vi "SUB_Write_GEN4_Init_data_V2_0_1 - 88.vi"(5 "Interval Time":enum16{"10ms", "33ms", "50ms"}(ring), 7 "Mode":T3, 8 "Connection Status":T1={"MAC Address"="F8:B8:54:EF:76:8D", "cnx handle"=0, "cnx flags"=5, "Address Type"=1, "Connection Interval (ms)"=8, "Timeout(ms)"=1000, "Latency"=0, "bonding handle"=255} {"Address Type" items=["Public", "Random"]}, 9 "88 tx start":bool, 10 "PCAP zero information":T4 {"Check sum" format="%x"; "Sensor 8_L" format="%x"; "Sensor 8_H" format="%x"; "Sensor 7_L" format="%x"; "Sensor 7_H" format="%x"; "Sensor 6_L" format="%x"; "Sensor 6_H" format="%x"; "Sensor 5_L" format="%x"; "Sensor 5_H" format="%x"; "Sensor 4_L" format="%x"; "Sensor 4_H" format="%x"; "Sensor 3_L" format="%x"; "Sensor 3_H" format="%x"; "Sensor 2_L" format="%x"; "Sensor 2_H" format="%x"; "Sensor 1_L" format="%x"; "Sensor 1_H" format="%x"; "Packet ID" format="%x"}, 11 "Port-act 1":refnum<visa-resource-name>="COM8") -> (0 "88 checksum":u8, 1 "88 rx start":bool)   [LabVIEW 2015]
uses:
  Cluster Type/PCAP zero information.ctl
  Type definition/write_mode.ctl
  Lib_Bled112 toolkit/type_def/connection_status_bundle.ctl
  Lib_Bled112 toolkit/type_def/address_type.ctl
  Lib_Bled112 toolkit/ble_functions/ble_write_by_handle_uint8array.vi
panel:
  in  "Delay(ms)":u32=3
  # "=> Sensor Offset Valure"
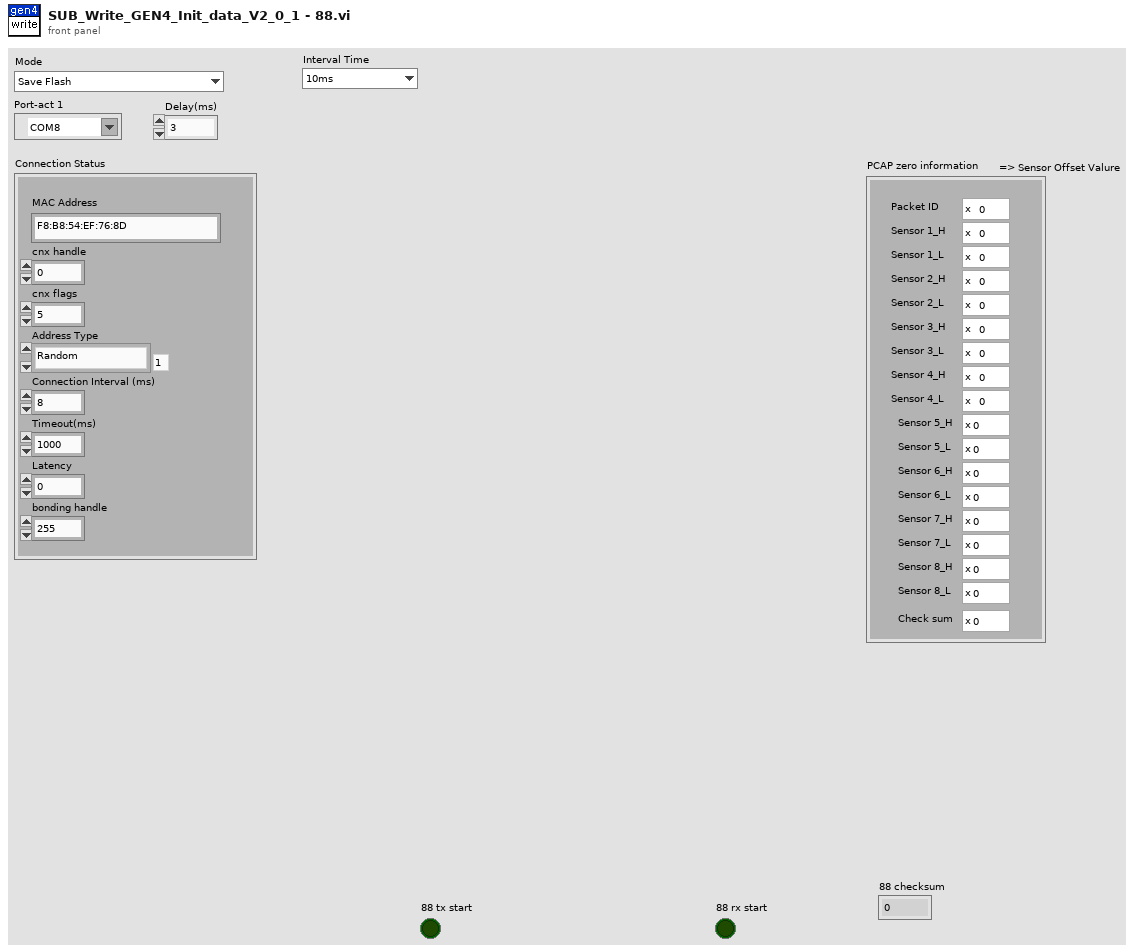
[diagram p1: front panel]
types:
  T1 = typedef "connection_status_bundle.ctl" = cluster{"MAC Address":string, "cnx handle":u8, "cnx flags":u8, "Address Type":T2, "Connection Interval (ms)":u16, "Timeout(ms)":u16, "Latency":u16, "bonding handle":u8}
  T2 = typedef "address_type.ctl" = u8
  T3 = typedef "write_mode.ctl" = enum16{"Save Flash", "Visa save", "Interval Change"}
  T4 = typedef "PCAP zero information.ctl" = cluster{"Packet ID":u8, "Sensor 1_H":u8, "Sensor 1_L":u8, "Sensor 2_H":u8, "Sensor 2_L ":u8, "Sensor 3_H":u8, "Sensor 3_L":u8, "Sensor 4_H":u8, "Sensor 4_L":u8, "Sensor 5_H":u8, "Sensor 5_L":u8, "Sensor 6_H":u8, "Sensor 6_L":u8, "Sensor 7_H":u8, "Sensor 7_L":u8, "Sensor 8_H":u8, "Sensor 8_L":u8, "Check sum":u8}
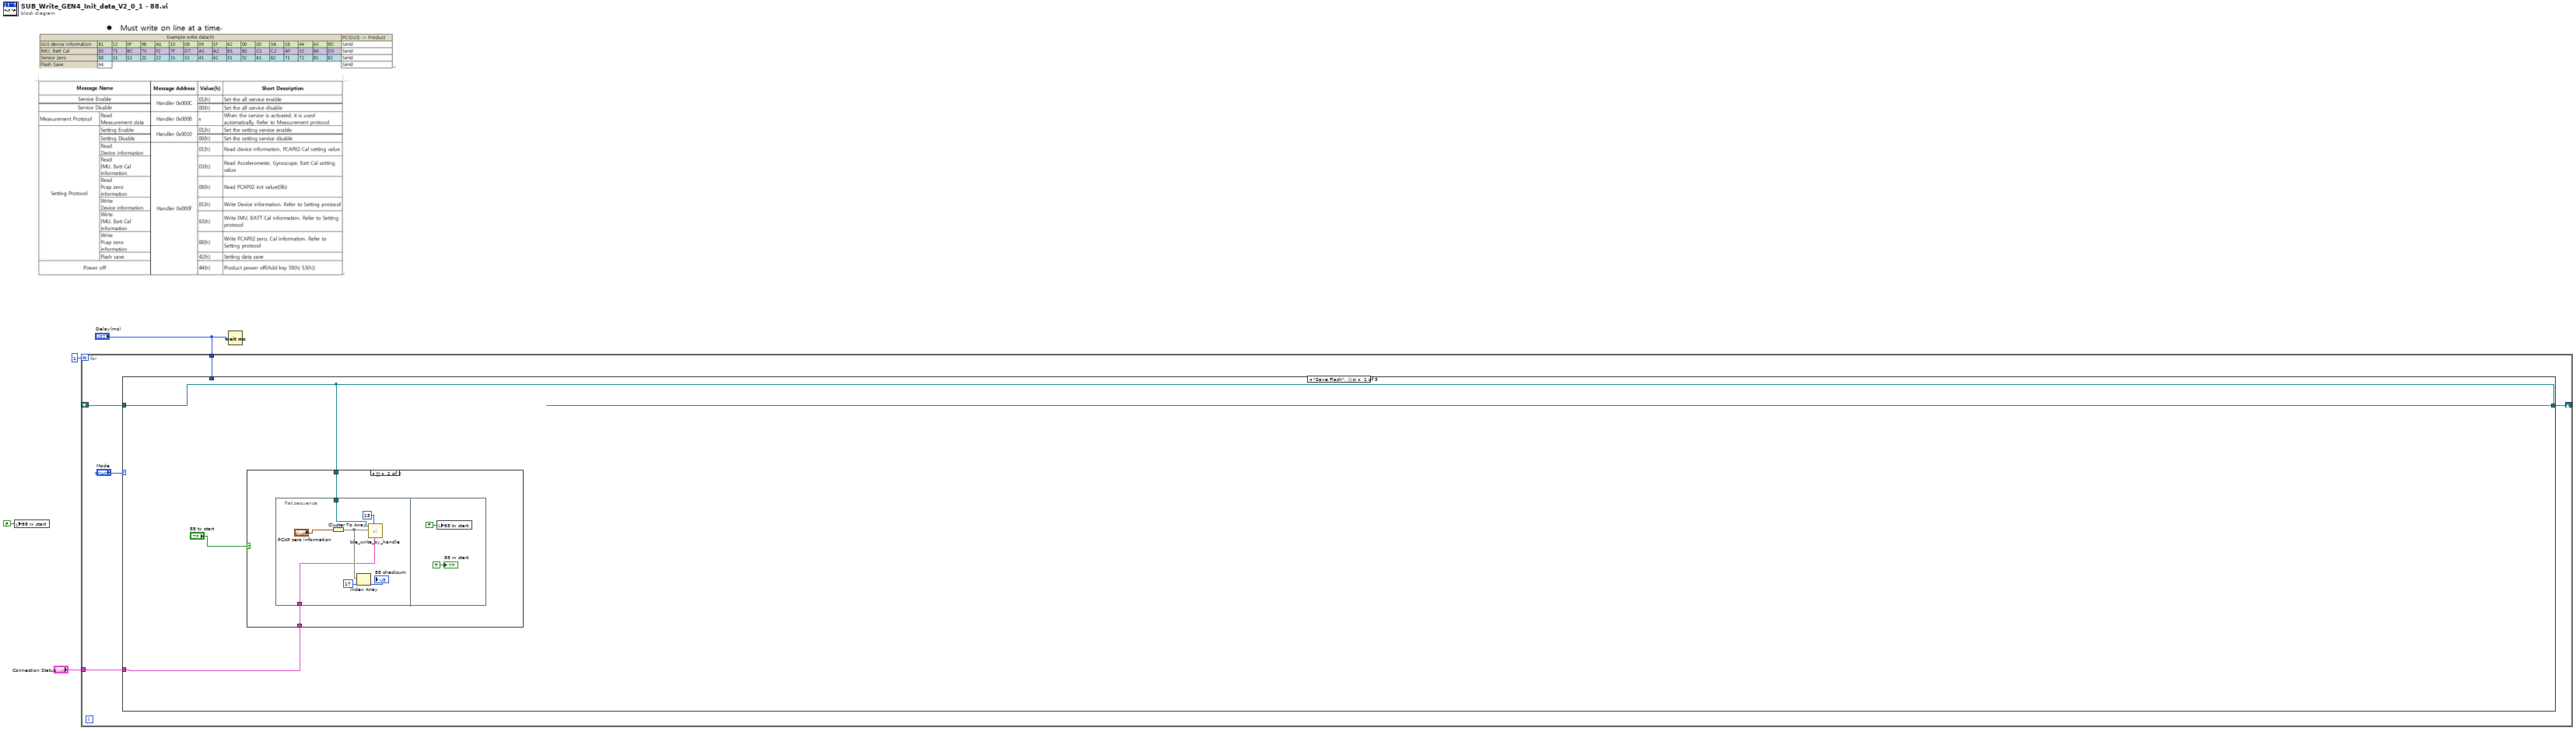
[diagram p0: block diagram]
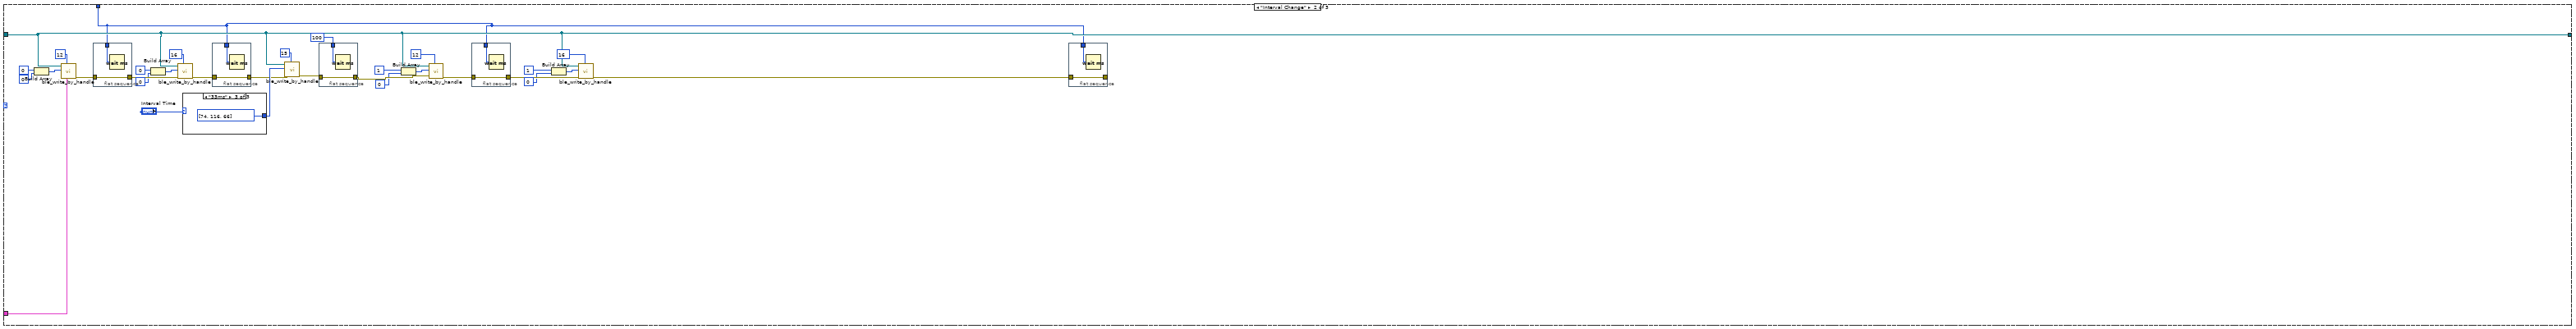
[diagram p3: hidden frame]
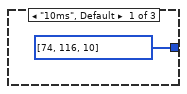
[diagram p4: hidden frame]
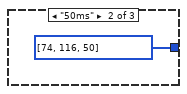
[diagram p5: hidden frame]
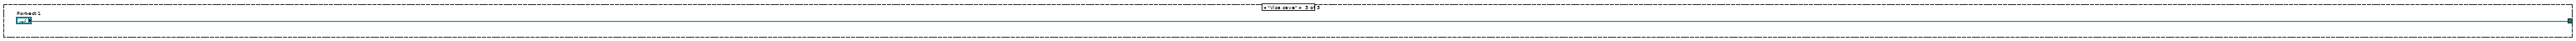
[diagram p6: hidden frame]
diagram:
  n1 = local write "88 rx start"(FALSE ("42 rx start")) -> ()
  n2 = for {
    N: 1 -> [_]
    shift-right: [w8] -> _
    shift-left: _ -> [w7]
    tunnel: "Connection Status" -> [w6]
    tunnel: "Delay(ms)" -> [w5]
    n3 = case shown="\"Save Flash\", 기본" "Mode" {
      tunnel: [w12 w41 "Port-act 1"] -> w8
      tunnel: w7 -> [w12 w41 _]
      tunnel: w6 -> [w11 w54 _]
      tunnel: w5 -> [_ w29 _]
      frame "Save Flash", Default {
        n4 = case shown="참" "88 tx start" {
          tunnel: w12 -> [_ w14]
          tunnel: w11 -> [_ w13]
          frame False {
          }
          frame True {
            n5 = flat-sequence {
              tunnel: w14 -> [w17]
              tunnel: w13 -> [w16]
              frame #0 {
                n6 = Cluster To Array(cluster="PCAP zero information") -> (array=w18:u8[])
                n7 = Index Array(array=w18, index=17 ("인덱스")) -> (element=→"88 checksum":u8)
                n8 = call-poly "ble_write_by_handle.vi"("Connection Status"=w16, "Handle"=u16 15, "data (uint8array)"=w18, "COM Bluegiga in"=w17) -> ()  [unwired: 6 in, 2 out]
              }
              frame #1 {
                n9 = local write "88 tx start"(FALSE ("88 tx start")) -> ()
                "88 rx start" <- TRUE ("42 rx start")
              }
            }
          }
        }
      }
      frame "Interval Change" {
        n10 = Build Array(u16 0 ("Handle"), u16 0 ("Handle")) -> (w52:u16[])
        n11 = call-poly "ble_write_by_handle.vi"("Connection Status"=w54, "Handle"=u16 12, "data (uint8array)"=w52, "COM Bluegiga in"=w41) -> ("error out"=w37:errorcluster)  [unwired: 6 in, 1 out]
        n12 = flat-sequence {
          tunnel: w29 -> [w65]
          tunnel: [w64] -> w38
          tunnel: w37 -> [w64]
          frame #0 {
            n13 = Wait (ms)(milliseconds to wait=w65) -> ()  [unwired: 1 out]
          }
        }
        n14 = Build Array(u16 0 ("Handle"), u16 0 ("Handle")) -> (w51:u16[])
        n15 = call-poly "ble_write_by_handle.vi"("Handle"=u16 16, "error in (no error)"=w38, "data (uint8array)"=w51, "COM Bluegiga in"=w41) -> ("error out"=w36:errorcluster)  [unwired: 6 in, 1 out]
        n16 = case shown="\"33ms\"" "Interval Time" {
          tunnel: [u8[] [74, 116, 10] u8[] [74, 116, 50] u8[] [74, 116, 66]] -> w39
          frame "10ms", Default {
          }
          frame "50ms" {
          }
          frame "33ms" {
          }
        }
        n17 = flat-sequence {
          tunnel: w29 -> [w63]
          tunnel: [w62] -> w35
          tunnel: w36 -> [w62]
          frame #0 {
            n18 = Wait (ms)(milliseconds to wait=w63) -> ()  [unwired: 1 out]
          }
        }
        n19 = call-poly "ble_write_by_handle.vi"("Handle"=u16 15, "error in (no error)"=w35, "data (uint8array)"=w39, "COM Bluegiga in"=w41) -> ("error out"=w34:errorcluster)  [unwired: 6 in, 1 out]
        n20 = flat-sequence {
          tunnel: u32 100 ("대기 시간(ms)") -> [w61]
          tunnel: [w60] -> w33
          tunnel: w34 -> [w60]
          frame #0 {
            n21 = Wait (ms)(milliseconds to wait=w61) -> ()  [unwired: 1 out]
          }
        }
        n22 = Build Array(u16 1 ("Handle"), u16 0 ("Handle")) -> (w45:u16[])
        n23 = call-poly "ble_write_by_handle.vi"("Handle"=u16 12, "error in (no error)"=w33, "data (uint8array)"=w45, "COM Bluegiga in"=w41) -> ("error out"=w32:errorcluster)  [unwired: 6 in, 1 out]
        n24 = flat-sequence {
          tunnel: w29 -> [w59]
          tunnel: [w58] -> w31
          tunnel: w32 -> [w58]
          frame #0 {
            n25 = Wait (ms)(milliseconds to wait=w59) -> ()  [unwired: 1 out]
          }
        }
        n26 = Build Array(u16 1 ("Handle"), u16 0 ("Handle")) -> (w46:u16[])
        n27 = call-poly "ble_write_by_handle.vi"("Handle"=u16 16, "error in (no error)"=w31, "data (uint8array)"=w46, "COM Bluegiga in"=w41) -> ("error out"=w30:errorcluster)  [unwired: 6 in, 1 out]
        n28 = flat-sequence {
          tunnel: w29 -> [w57]
          tunnel: [w56] -> _
          tunnel: w30 -> [w56]
          frame #0 {
            n29 = Wait (ms)(milliseconds to wait=w57) -> ()  [unwired: 1 out]
          }
        }
      }
      frame "Visa save" {
      }
    }
  }
  n30 = Wait (ms)(milliseconds to wait="Delay(ms)") -> ()  [unwired: 1 out]
